vi "WF - Append Src Name to Sig Name.vi"(0 "wForm IN":waveform(dbl), 5 "error in (no error)":errorcluster) -> (14 "wForm OUT":waveform(dbl), 19 "error out":errorcluster)   [LabVIEW 2022 SP3, in "GSwFormDSP.lvclass"]
uses:
  GSwFormDSP.lvclass
  functions/Attribute List.ctl
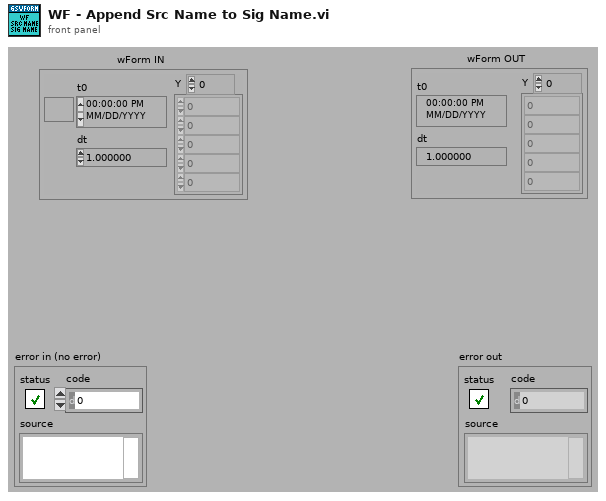
[diagram p1: front panel]
types:
  T1 = typedef "GSwFormDSP.lvclass/Attribute List.ctl" = string
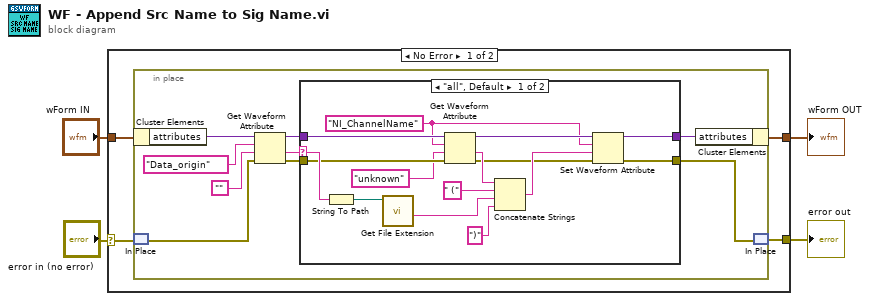
[diagram p0: block diagram]
diagram:
  n1 = case shown="No Error" "error in (no error)" {
    selector: "error in (no error)" -> [w7 w36]
    tunnel: [w5 w36] -> w3
    tunnel: [w6 w35] -> w1
    tunnel: "wForm IN" -> [w8 w35]
    frame No Error {
      n2 = in-place {
        n3 = in-place-cluster #1(w8) -> ("attributes"=w17:variant)
        n4 = in-place-match #2(w7) -> (w11:errorcluster)
        n5 = Get Waveform Attribute(4:w11, 5:"", 6:T1 "Data_origin" ("wForm Attributes"), 7:w17) -> (0:w10:errorcluster, 1:w14:string, 3:w12:variant)  [unwired: 1 out]
        n6 = case shown="\"all\", Default" w14 {
          selector: w14 -> [w32 _]
          tunnel: [w23 w34] -> w13
          tunnel: w12 -> [w30 w34]
          tunnel: w10 -> [w29 w33]
          tunnel: [w18 w33] -> w9
          frame "all", Default {
            w21 = T1 "NI_ChannelName" ("wForm Attributes")
            n7 = String To Path(string=w32) -> (path=w31:path)
            n8 = call <vilib>:"Get File Extension.vi"("file"=w31) -> ("filename without extension"=w25:string)  [unwired: 6 in, 4 out]
            n9 = Get Waveform Attribute(4:w29, 5:"unknown", 6:w21, 7:w30) -> (0:w19:errorcluster, 1:w27:string, 3:w22:variant)  [unwired: 1 out]
            n10 = Concatenate Strings(w27, " (" ("string"), w25, ")") -> (w20:string)
            n11 = Set Waveform Attribute(4:w19, 5:w20, 6:w21, 7:w22) -> (0:w18:errorcluster, 3:w23:variant)  [unwired: 1 out]
          }
          frame "" {
            # "Empty Source, so do nothing."
          }
        }
        n12 = in-place-cluster #1("attributes"=w13) -> (w6:waveform(dbl))
        n13 = in-place-match #2(w9) -> (w5:errorcluster)
      }
    }
    frame Error {
    }
  }
  "error out" <- w3
  "wForm OUT" <- w1
